vi "Test Add Multiple Methods in Different Cases.vi"(8 "error in (no error)":errorcluster, 11 "Result Model Tests in":refnum<class "Result Model Tests.lvclass">) -> (0 "error out":errorcluster, 3 "Result Model Tests out":refnum<class "Result Model Tests.lvclass">)   [LabVIEW 2020, in "Result Model Tests.lvclass"]
uses:
  Result Model Tests.lvclass
  Result Model Tests.lvclass/Result Model Tests.ctl
  Result Model/Result Model.lvclass
  206db1ee-aa99-40b9-8881-171f2a77c34b.vi
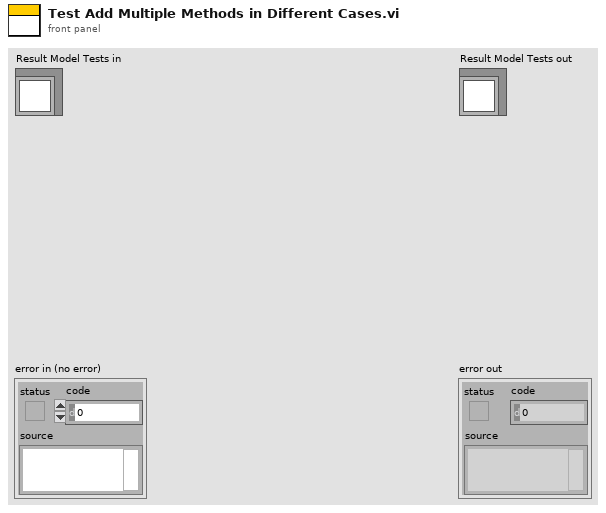
[diagram p1: front panel]
types:
  T1 = cluster{"Left Cell String":string, "Child Text":string[], "Child Tag":string, "Item Indent":i32, "Child Only?":bool, "Glyph Index":i32}[]
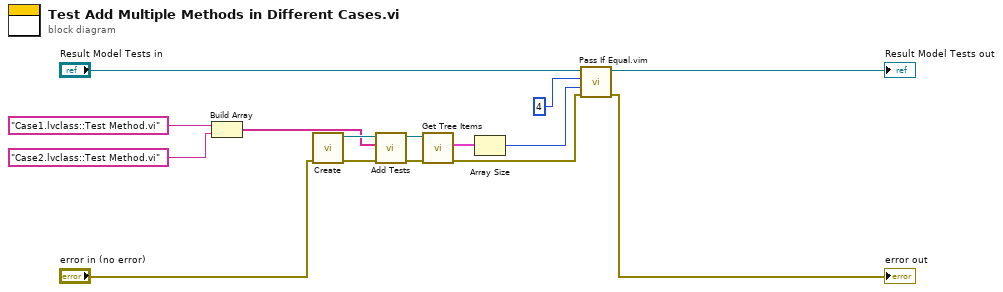
[diagram p0: block diagram]
diagram:
  n1 = Build Array("Case1.lvclass::Test Method.vi" ("String"), "Case2.lvclass::Test Method.vi" ("String")) -> (w8:string[])
  n2 = call "Create.vi"("error in (no error)"="error in (no error)") -> ("error out"=w13:errorcluster, "Result Model out"=w14:refnum<class "Result Model.lvclass">)  [unwired: 9 in]
  n3 = call "Add Tests.vi"("error in (no error)"=w13, "Tests"=w8, "Result Model In"=w14) -> ("error out"=w11:errorcluster, "Result Model Out"=w12:refnum<class "Result Model.lvclass">)  [unwired: 7 in]
  n4 = call "Get Tree Items.vi"("error in (no error)"=w11, "Result Model In"=w12) -> ("error out"=w6:errorcluster, "Tree Items"=w3:T1)  [unwired: 7 in, 1 out]
  n5 = Array Size(array=w3) -> (size(s)=w2:i32)
  n6 = call "Pass If Equal.vim"("error in (no error)"=w6, "Actual"=w2, "Expected"=4 ("size(s)"), "LUnit Test Case In"="Result Model Tests in") -> ("error out"=→"error out":errorcluster, "LUnit Test Case Out"=→"Result Model Tests out":refnum<class "Result Model Tests.lvclass">)  [unwired: 6 in]
